vi "Write JSON Prop.vi"(7 "JSON Path":string, 8 "error in (no error)":errorcluster, 10 "Value":variant, 11 "Ctl Refnum in":refnum<vi>) -> (0 "error out":errorcluster, 3 "Ctl Refnum":refnum<vi>)   [LabVIEW 2020, in "VolatusGUIEditorCore.lvlib"]
uses:
  VolatusGUIEditorCore.lvlib
  VolatusGUIControls/VolatusGUIControls.lvlib
  7578c3fd-306e-425c-88c0-b516f66cc273.vi
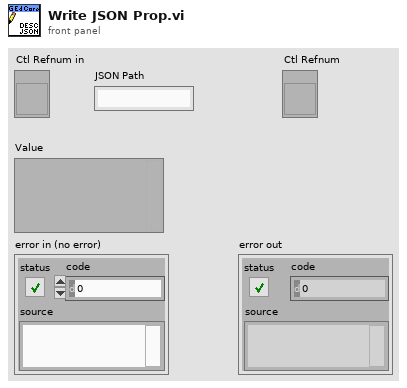
[diagram p1: front panel]
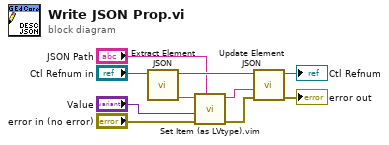
[diagram p0: block diagram]
diagram:
  n1 = call "Extract Element JSON.vi"("Ctl Refnum in"="Ctl Refnum in") -> ("JSON"=w10:string, "Ctl Refnum"=w9:refnum<vi>)  [unwired: 7 in, 2 out]
  n2 = call "Set Item (as LVtype).vim"("$Path or Item Name"="JSON Path", "error in (no error)"="error in (no error)", "Anything"="Value", "JSON"=w10) -> ("error out"=w7:errorcluster, "<JSON>"=w8:string)  [unwired: 4 in, 1 out]
  n3 = call "Update Element JSON.vi"("error in (no error)"=w7, "JSON"=w8, "Ctl Refnum in"=w9) -> ("error out"=→"error out":errorcluster, "Ctl Refnum"=→"Ctl Refnum":refnum<vi>)  [unwired: 7 in]
